vi "Global Mapper C.vi"(11 "GIC Input":T1={"     Use ?\nOff       On"=[FALSE, TRUE, FALSE, TRUE], "Mode:"=FALSE, "WP Data"="", "Hokuyo Port"="COM7", "Prop  Port"="COM6", "Compass Port"="", "GPS Port"="", "Num of WPs"=0, "WP Lats and Longs"={"WP Lats"=[], "WP Longs"=[]}, "Obst Lats and Longs"={"Obst Lats"=[], "Obst Longs"=[]}, "Parameters"=[], "GPS Data"=[], "Compass"=0.0, "LMS Vector"=[], "Vision Vector"=[], "Direction Cmd"=0.0, "Speed Cmd"=0.0, "WP Vector"=[], "WP Number"=0, "Extra"=0, "SW Map"=[], "Path Cluster"={"Path x node"=[], "Path y node"=[]}} {"Obst Lats and Longs"."Obst Longs" format="%#_8g"; "Obst Lats and Longs"."Obst Lats" format="%#_8g"}) -> (3 "Picture with Robot and WPs and Obstacles":picture)   [LabVIEW 2014]
panel:
  # "Global Mapper C"
  # "Input:"
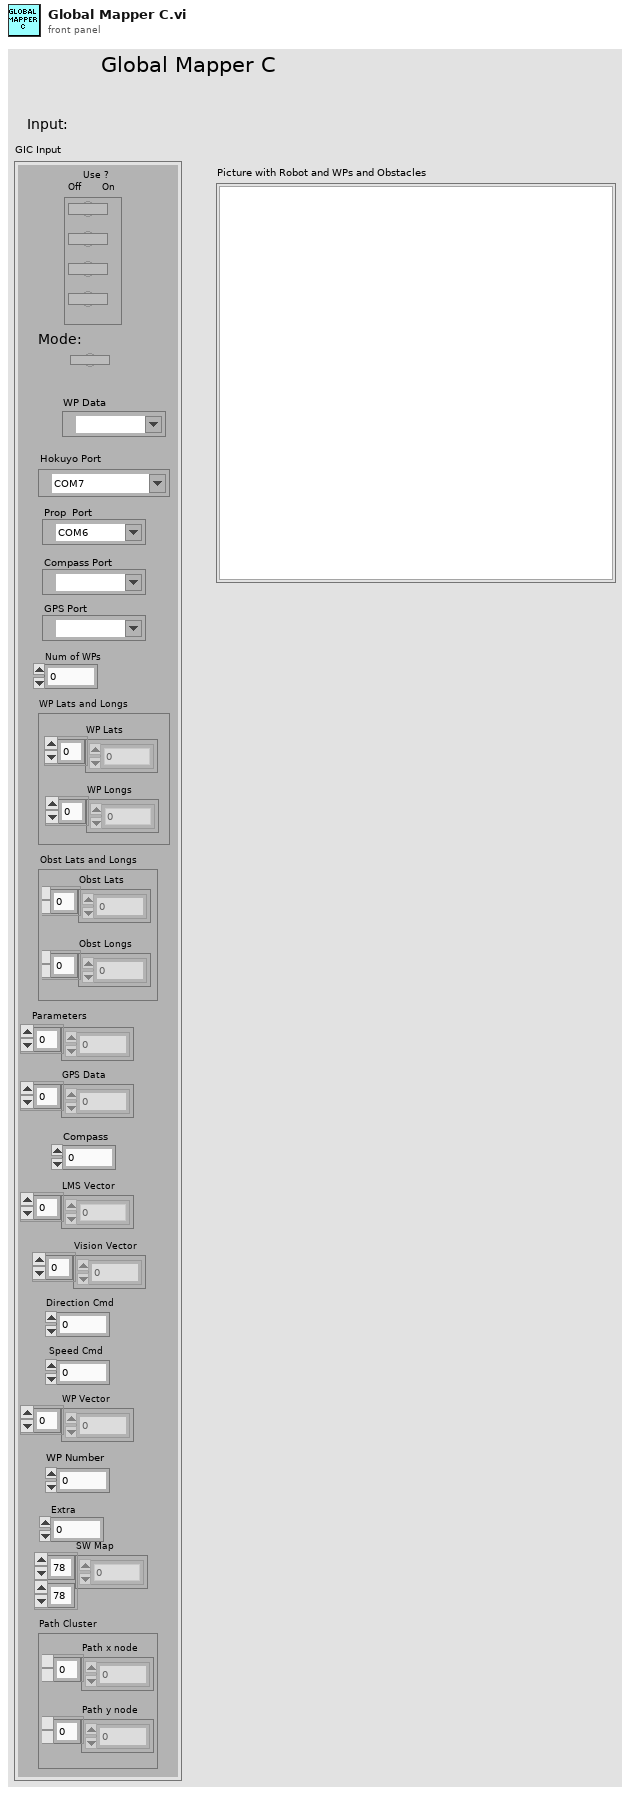
[diagram p1: front panel]
types:
  T1 = cluster{"     Use ?\nOff       On":bool[], "Mode:":bool, "WP Data":refnum<visa-resource-name>, "Hokuyo Port":refnum<visa-resource-name>, "Prop  Port":refnum<visa-resource-name>, "Compass Port":refnum<visa-resource-name>, "GPS Port":refnum<visa-resource-name>, "Num of WPs":i16, "WP Lats and Longs":cluster{"WP Lats":dbl[], "WP Longs":dbl[]}, "Obst Lats and Longs":cluster{"Obst Lats":dbl[], "Obst Longs":dbl[]}, "Parameters":dbl[], "GPS Data":dbl[], "Compass":dbl, "LMS Vector":dbl[], "Vision Vector":dbl[], "Direction Cmd":dbl, "Speed Cmd":dbl, "WP Vector":dbl[], "WP Number":i32, "Extra":i16, "SW Map":i32[][], "Path Cluster":cluster{"Path x node":dbl[], "Path y node":dbl[]}}
  T2 = cluster{"Width":u16, "Style":enum32{"Solid", "Dash", "Dot", "DashDot", "DashDotDot"}}
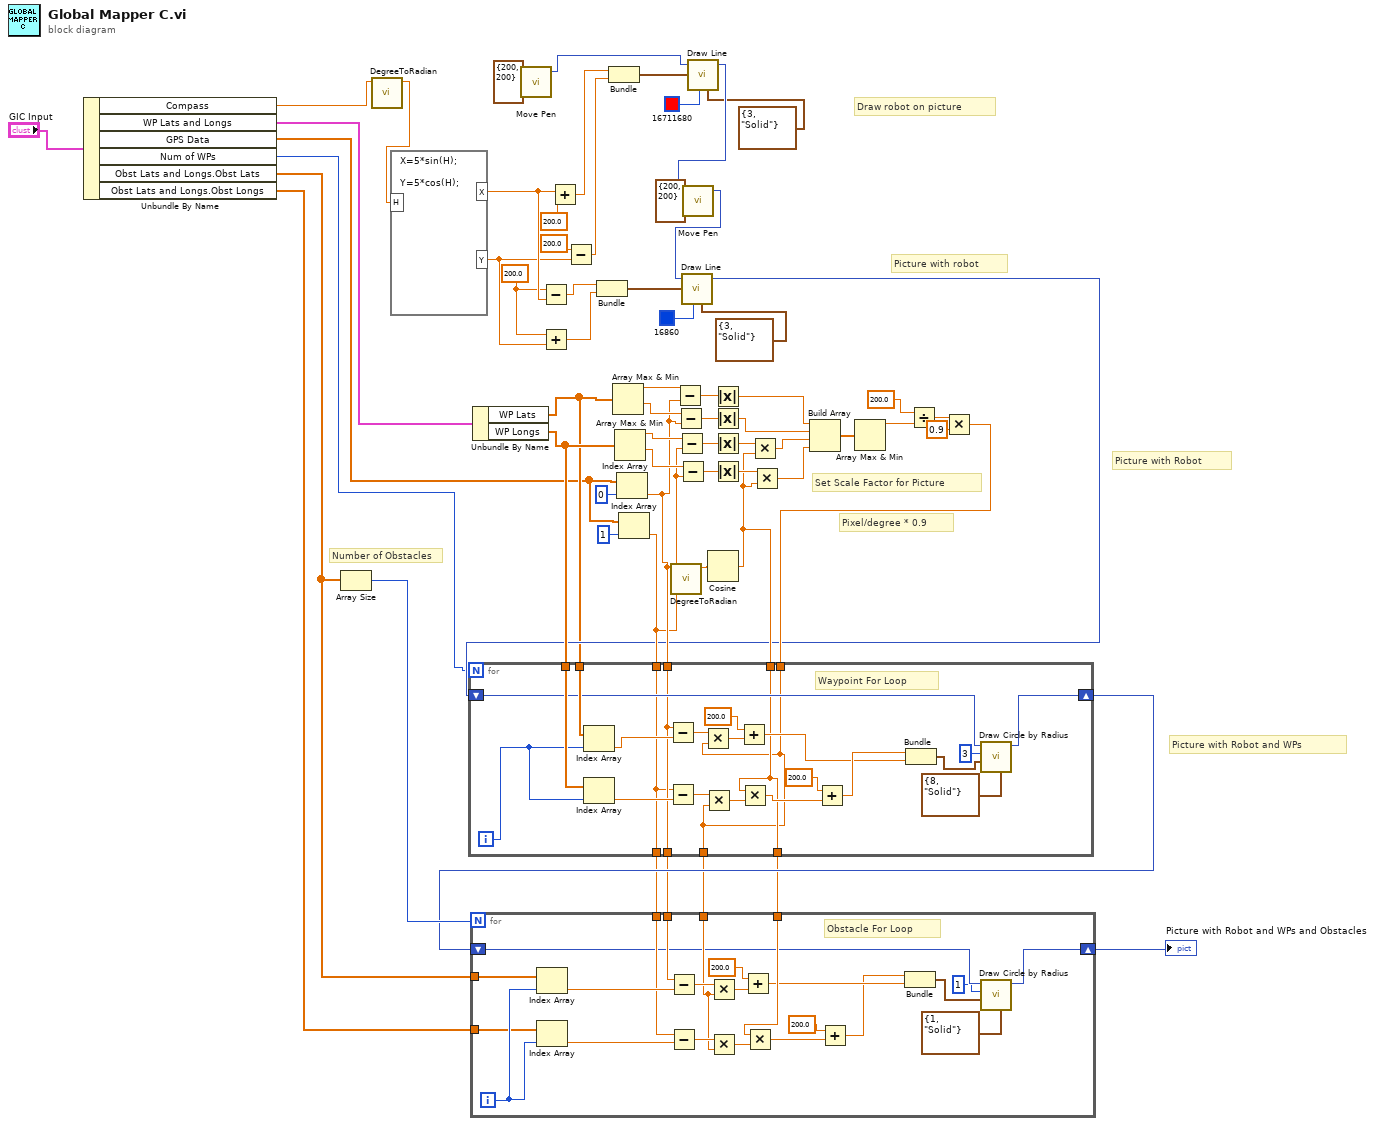
[diagram p0: block diagram]
diagram:
  w50 = 200.0 ("x")
  # "Picture with Robot and WPs"
  # "Picture with Robot"
  # "Number of Obstacles"
  # "Set Scale Factor for Picture"
  # "Pixel/degree * 0.9"
  # "Picture with robot"
  # "Draw robot on picture"
  n1 = Unbundle By Name("GIC Input") -> ("Compass"=w14:dbl, "WP Lats and Longs"=w13:cluster{"WP Lats":dbl[], "WP Longs":dbl[]}, "GPS Data"=w12:dbl[], "Num of WPs"=w11:i16, "Obst Lats and Longs.Obst Lats"=w7:dbl[], "Obst Lats and Longs.Obst Longs"=w6:dbl[])
  n2 = Array Size(array=w7) -> (size(s)=w9:i32)
  n3 = call "DegreeToRadian.vi"("Degrees"=w14) -> ("Radians"=w46:dbl)  [unwired: 10 in]
  n4 = formula code="X=5*sin(H);\n\nY=5*cos(H);"("H"=w46) -> ("X"=w52:dbl, "Y"=w49:dbl)
  n5 = Unbundle By Name(w13) -> ("WP Lats"=w15:dbl[], "WP Longs"=w20:dbl[])
  n6 = call <vilib>:"Move Pen.vi"("new position"=cluster{"x":i16, "y":i16} {"x"=200, "y"=200}) -> ("new picture"=w63:picture)  [unwired: 4 in]
  n7 = Subtract(x=w50, y=w52) -> (x-y=w51:dbl)
  n8 = Add(x=w50, y=w49) -> (x+y=w48:dbl)
  n9 = Add(x=w52, y=200.0) -> (x+y=w56:dbl)
  n10 = Subtract(x=200.0, y=w49) -> (x-y=w54:dbl)
  n11 = Bundle(w51, w48) -> (w47:cluster{dbl, dbl})  [unwired: 1 in]
  n12 = Bundle(w56, w54) -> (w53:cluster{dbl, dbl})  [unwired: 1 in]
  n13 = Array Max & Min(array=w15) -> (max value=w41:dbl, min value=w26:dbl)  [unwired: 2 out]
  n14 = Array Max & Min(array=w20) -> (max value=w38:dbl, min value=w35:dbl)  [unwired: 2 out]
  n15 = Index Array(array=w12, index=0) -> (element=w21:dbl)
  n16 = Index Array(array=w12, index=1) -> (element=w19:dbl)
  n17 = call "DegreeToRadian.vi"("Degrees"=w21) -> ("Radians"=w24:dbl)  [unwired: 10 in]
  n18 = Subtract(x=w41, y=w21) -> (x-y=w40:dbl)
  n19 = Subtract(x=w26, y=w21) -> (x-y=w39:dbl)
  n20 = Subtract(x=w38, y=w19) -> (x-y=w37:dbl)
  n21 = Subtract(x=w35, y=w19) -> (x-y=w34:dbl)
  n22 = call <vilib>:"Draw Line.vi"("picture"=w63, "end point"=w53, "color(black)"=u32 16711680, "pen"=T2 {"Width"=3, "Style"=enum."Solid"}) -> ("new picture"=w61:picture)  [unwired: 5 in]
  n23 = call <vilib>:"Move Pen.vi"("new position"=cluster{"x":i16, "y":i16} {"x"=200, "y"=200}, "picture"=w61) -> ("new picture"=w59:picture)  [unwired: 3 in]
  n24 = call <vilib>:"Draw Line.vi"("picture"=w59, "end point"=w47, "color(black)"=u32 16860, "pen"=T2 {"Width"=3, "Style"=enum."Solid"}) -> ("new picture"=w16:picture)  [unwired: 5 in]
  n25 = Cosine(x=w24) -> (cos(x)=w17:dbl)
  n26 = Absolute Value(x=w40) -> (abs(x)=w28:dbl)
  n27 = Absolute Value(x=w39) -> (abs(x)=w27:dbl)
  n28 = Absolute Value(x=w37) -> (abs(x)=w36:dbl)
  n29 = Absolute Value(x=w34) -> (abs(x)=w33:dbl)
  n30 = Multiply(x=w36, y=w17) -> (x*y=w32:dbl)
  n31 = Multiply(x=w33, y=w17) -> (x*y=w31:dbl)
  n32 = Build Array(w28, w27, w32, w31) -> (w30:dbl[])
  n33 = Array Max & Min(array=w30) -> (max value=w25:dbl)  [unwired: 3 out]
  n34 = Divide(x=200.0, y=w25) -> (x/y=w23:dbl)
  n35 = Multiply(x=w23, y=0.9) -> (x*y=w18:dbl)
  n36 = for {
    N: w11 -> [_]
    tunnel: w21 -> [w68]
    tunnel: w20 -> [w74]
    tunnel: w19 -> [w67]
    tunnel: w18 -> [w65]
    tunnel: w17 -> [w66]
    shift-right: [w80] -> w8
    shift-left: w16 -> [w69]
    tunnel: w15 -> [w73]
    tunnel: [w68] -> w5
    tunnel: [w67] -> w4
    tunnel: [w66] -> w3
    tunnel: [w65] -> w2
    i -> [w70]
    # "Waypoint For Loop"
    n37 = Index Array(array=w73, index=w70) -> (element=w72:dbl)
    n38 = Index Array(array=w74, index=w70) -> (element=w71:dbl)
    n39 = Subtract(x=w68, y=w72) -> (x-y=w87:dbl)
    n40 = Subtract(x=w67, y=w71) -> (x-y=w84:dbl)
    n41 = Multiply(x=w87, y=w65) -> (x*y=w86:dbl)
    n42 = Multiply(x=w84, y=w65) -> (x*y=w82:dbl)
    n43 = Add(x=200.0, y=w86) -> (x+y=w75:dbl)
    n44 = Multiply(x=w66, y=w82) -> (x*y=w81:dbl)
    n45 = Add(x=200.0, y=w81) -> (x+y=w76:dbl)
    n46 = Bundle(w76, w75) -> (w78:cluster{dbl, dbl})  [unwired: 1 in]
    n47 = call <vilib>:"Draw Circle by Radius.vi"("pen"=T2 {"Width"=8, "Style"=enum."Solid"}, "pixel center"=w78, "radius"=i16 3, "picture"=w69) -> ("new picture"=w80:picture)  [unwired: 7 in]
  }
  n48 = for {
    N: w9 -> [_]
    shift-right: [w91] -> w1
    shift-left: w8 -> [w92]
    tunnel: w7 -> [w110]
    tunnel: w6 -> [w108]
    tunnel: w5 -> [w107]
    tunnel: w4 -> [w105]
    tunnel: w3 -> [w96]
    tunnel: w2 -> [w95]
    i -> [w109]
    # "Obstacle For Loop"
    n49 = Index Array(array=w110, index=w109) -> (element=w106:dbl)
    n50 = Index Array(array=w108, index=w109) -> (element=w104:dbl)
    n51 = Subtract(x=w107, y=w106) -> (x-y=w103:dbl)
    n52 = Subtract(x=w105, y=w104) -> (x-y=w100:dbl)
    n53 = Multiply(x=w103, y=w95) -> (x*y=w102:dbl)
    n54 = Multiply(x=w100, y=w95) -> (x*y=w99:dbl)
    n55 = Add(x=200.0, y=w102) -> (x+y=w94:dbl)
    n56 = Multiply(x=w96, y=w99) -> (x*y=w98:dbl)
    n57 = Add(x=200.0, y=w98) -> (x+y=w93:dbl)
    n58 = Bundle(w93, w94) -> (w89:cluster{dbl, dbl})  [unwired: 1 in]
    n59 = call <vilib>:"Draw Circle by Radius.vi"("pen"=T2 {"Width"=1, "Style"=enum."Solid"}, "pixel center"=w89, "radius"=i16 1, "picture"=w92) -> ("new picture"=w91:picture)  [unwired: 7 in]
  }
  "Picture with Robot and WPs and Obstacles" <- w1
